vi "3.3.1.-SubVI Conversión RGB a HSV.vi"(9 "B":u8, 10 "G":u8, 11 "R":u8) -> (1 "S":dbl, 2 "H":dbl, 4 "V":dbl)   [LabVIEW 2020]
panel:
  # "Visión Artificial - Convertir Capas RGB a HSV\nDiego Cervantes Rodríguez\ndicer0.com"
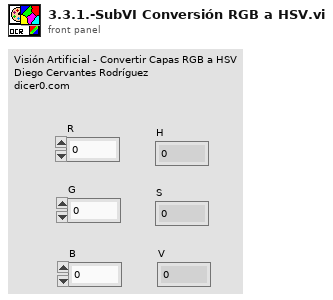
[diagram p1: front panel]
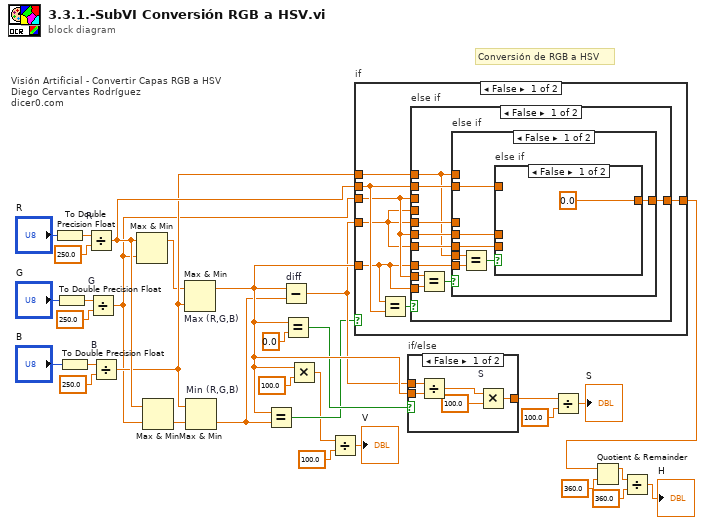
[diagram p0: block diagram]
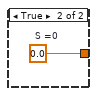
[diagram p2: hidden frame]
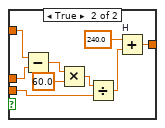
[diagram p3: hidden frame]
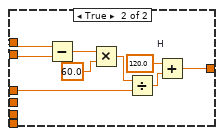
[diagram p4: hidden frame]
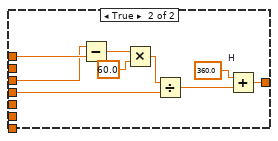
[diagram p5: hidden frame]
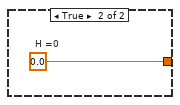
[diagram p6: hidden frame]
diagram:
  # "Visión Artificial - Convertir Capas RGB a HSV\nDiego Cervantes Rodríguez\ndicer0.com"
  # "Conversión de RGB a HSV"
  n1 = To Double Precision Float(number="R") -> (double precision float=w9:dbl)
  n2 = To Double Precision Float(number="G") -> (double precision float=w10:dbl)
  n3 = To Double Precision Float(number="B") -> (double precision float=w13:dbl)
  n4 = Divide "R"(x=w9, y=250.0) -> (x/y=w29:dbl)
  n5 = Divide "G"(x=w10, y=250.0) -> (x/y=w26:dbl)
  n6 = Divide "B"(x=w13, y=250.0) -> (x/y=w27:dbl)
  n7 = Max & Min(x=w29, y=w26) -> (max(x,y)=w18:dbl)  [unwired: 1 out]
  n8 = Max & Min(x=w29, y=w26) -> (min(x,y)=w19:dbl)  [unwired: 1 out]
  n9 = Max & Min "Max (R,G,B)"(x=w18, y=w27) -> (max(x,y)=w32:dbl)  [unwired: 1 out]
  n10 = Max & Min "Min (R,G,B)"(x=w27, y=w19) -> (min(x,y)=w23:dbl)  [unwired: 1 out]
  n11 = Equal?(x=w32, y=w23) -> (x = y?=w22:bool)
  n12 = Subtract "diff"(x=w32, y=w23) -> (x-y=w28:dbl)
  n13 = Equal?(x=w32, y=0.0) -> (x = y?=w24:bool)
  n14 = Multiply(x=w32, y=100.0) -> (x*y=w21:dbl)
  n15 = Divide(x=w21, y=100.0) -> (x/y=→"V":dbl)
  n16 = case "if" shown="False" w22 {
    tunnel: [w34 w85] -> w30
    tunnel: w26 -> [w36 _]
    tunnel: w27 -> [w39 _]
    tunnel: w28 -> [w35 _]
    tunnel: w32 -> [w33 _]
    tunnel: w29 -> [w37 _]
    frame False {
      n17 = Equal?(x=w33, y=w37) -> (x = y?=w38:bool)
      n18 = case "else if" shown="False" w38 {
        tunnel: w36 -> [_ w78]
        tunnel: w39 -> [w42 w83]
        tunnel: w35 -> [_ w77]
        tunnel: w33 -> [w40 _]
        tunnel: w36 -> [w41 _]
        tunnel: w37 -> [w48 _]
        tunnel: w35 -> [w47 _]
        tunnel: w36 -> [w46 _]
        tunnel: w35 -> [w45 _]
        tunnel: [w44 w76] -> w34
        tunnel: w33 -> [w43 _]
        frame False {
          n19 = Equal?(x=w41, y=w40) -> (x = y?=w49:bool)
          n20 = case "else if" shown="False" w49 {
            tunnel: w42 -> [_ w70]
            tunnel: w48 -> [w56 w69]
            tunnel: w47 -> [_ w68]
            tunnel: w46 -> [w55 _]
            tunnel: w45 -> [w54 _]
            tunnel: [w53 w67] -> w44
            tunnel: w43 -> [w50 _]
            tunnel: w42 -> [w51 _]
            frame False {
              n21 = Equal?(x=w51, y=w50) -> (x = y?=w52:bool)
              n22 = case "else if" shown="False" w52 {
                tunnel: w56 -> [_ w61]
                tunnel: w55 -> [_ w60]
                tunnel: w54 -> [_ w59]
                tunnel: [0.0 w58] -> w53
                frame False {
                }
                frame True {
                  n23 = Subtract(x=w61, y=w60) -> (x-y=w64:dbl)
                  n24 = Multiply(x=w64, y=60.0) -> (x*y=w65:dbl)
                  n25 = Divide(x=w65, y=w59) -> (x/y=w66:dbl)
                  n26 = Add "H"(x=240.0, y=w66) -> (x+y=w58:dbl)
                }
              }
            }
            frame True {
              n27 = Subtract(x=w70, y=w69) -> (x-y=w74:dbl)
              n28 = Multiply(x=w74, y=60.0) -> (x*y=w73:dbl)
              n29 = Divide(x=w73, y=w68) -> (x/y=w72:dbl)
              n30 = Add "H"(x=120.0, y=w72) -> (x+y=w67:dbl)
            }
          }
        }
        frame True {
          n31 = Subtract(x=w78, y=w83) -> (x-y=w82:dbl)
          n32 = Multiply(x=w82, y=60.0) -> (x*y=w81:dbl)
          n33 = Divide(x=w81, y=w77) -> (x/y=w80:dbl)
          n34 = Add "H"(x=360.0, y=w80) -> (x+y=w76:dbl)
        }
      }
    }
    frame True {
      w85 = 0.0  # H =0
    }
  }
  n35 = case "if/else" shown="False" w24 {
    tunnel: [w86 w91] -> w31
    tunnel: w28 -> [w90 _]
    tunnel: w32 -> [w89 _]
    frame False {
      n36 = Divide(x=w90, y=w89) -> (x/y=w87:dbl)
      n37 = Multiply "S"(x=w87, y=100.0) -> (x*y=w86:dbl)
    }
    frame True {
      w91 = 0.0  # S =0
    }
  }
  n38 = Divide(x=w31, y=100.0) -> (x/y=→"S":dbl)
  n39 = Quotient & Remainder(x=w30, y=360.0) -> (x-y*floor(x/y)=w3:dbl)  [unwired: 1 out]
  n40 = Divide(x=w3, y=360.0) -> (x/y=→"H":dbl)
